vi "avg_spectrum_gen.vi"(0 "IR_off_q_in":refnum<queue>, 1 "IR_off_q_error_in":errorcluster, 2 "IR_on_q_in":refnum<queue>, 3 "IR_on_q_error_in":errorcluster, 4 "power_q_in":refnum<queue>, 5 "power_q_error_in":errorcluster, 6 "Number of sweeps":dbl) -> (7 "Avg Off Trace":waveform(dbl), 8 "Off queue length":i32, 9 "Avg On Trace":waveform(dbl), 10 "On queue length":i32, 11 "Difference Trace":waveform(dbl), 12 "Finished Gathering":bool, 13 "Avg Power / J":dbl format="%#_6f", 14 "IR_off_q_out":refnum<queue>, 15 "IR_off_q_error_out":errorcluster, 16 "IR_on_q_out":refnum<queue>, 17 "IR_on_q_error_out":errorcluster, 18 "power_q_out":refnum<queue>, 19 "power_q_error_out":errorcluster)   [LabVIEW 2020]
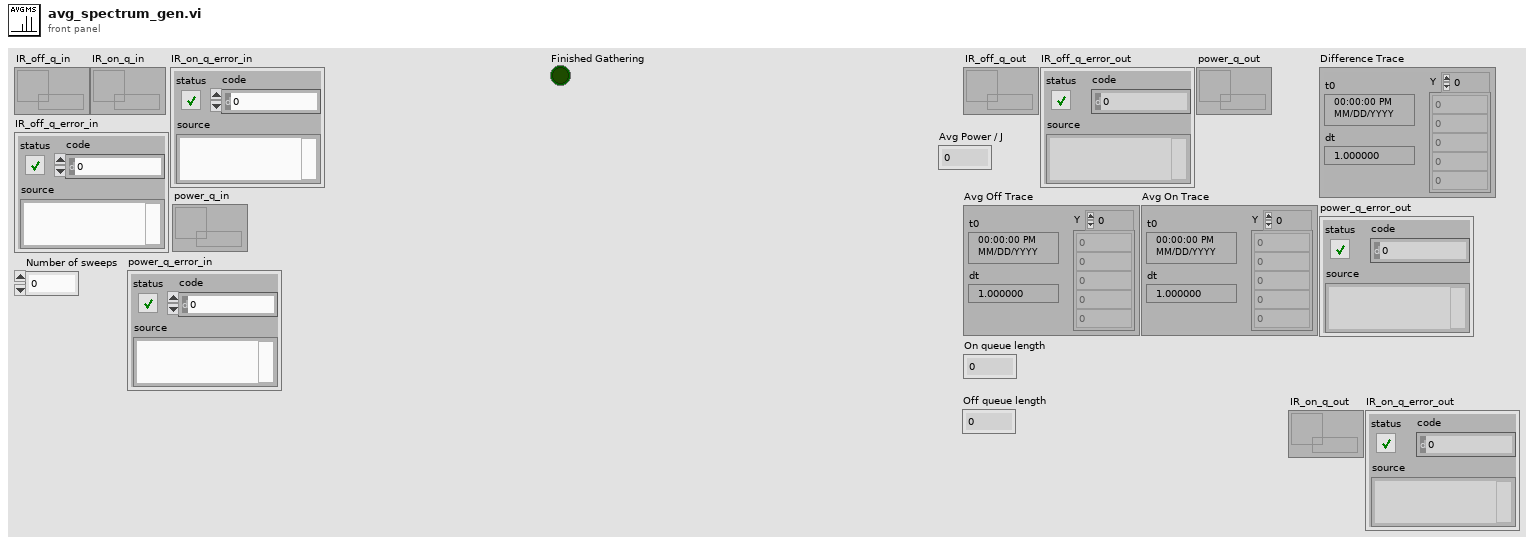
[diagram p1: front panel]
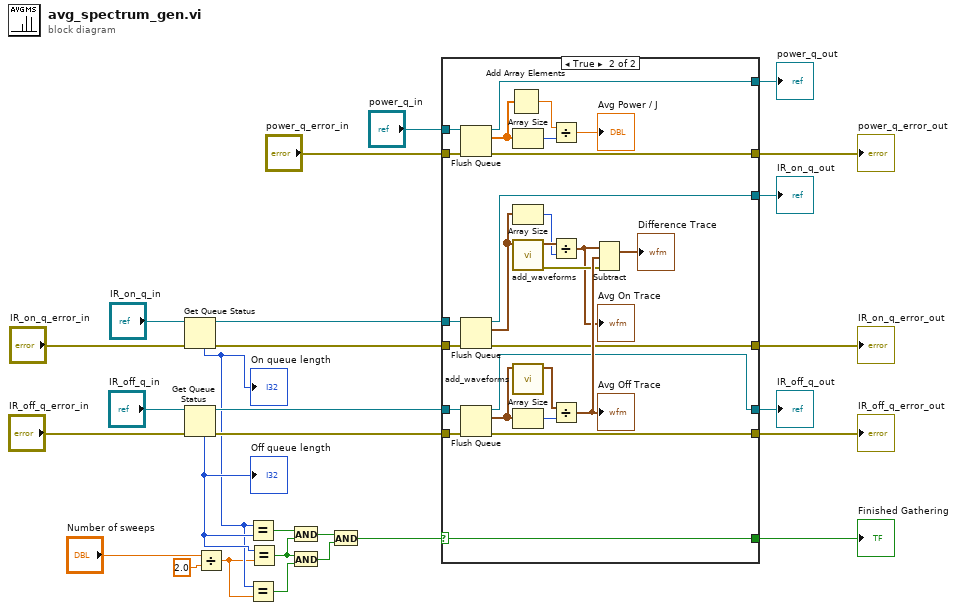
[diagram p0: block diagram]
diagram:
  n1 = Get Queue Status(queue="IR_on_q_in", error in (no error)="IR_on_q_error_in") -> (queue out=w24:refnum<queue>, error out=w23:errorcluster, # elements in queue=w14:i32)  [unwired: 1 in, 5 out]
  "On queue length" <- w14
  n2 = Get Queue Status(queue="IR_off_q_in", error in (no error)="IR_off_q_error_in") -> (queue out=w26:refnum<queue>, error out=w25:errorcluster, # elements in queue=w15:i32)  [unwired: 1 in, 5 out]
  "Off queue length" <- w15
  n3 = Divide(x="Number of sweeps", y=2.0) -> (x/y=w4:dbl)
  n4 = Equal?(x=w14, y=w15) -> (x = y?=w11:bool)
  n5 = Equal?(x=w14, y=w4) -> (x = y?=w9:bool)
  n6 = Equal?(x=w15, y=w4) -> (x = y?=w8:bool)
  n7 = And(x=w11, y=w8) -> (x .and. y?=w10:bool)
  n8 = And(x=w8, y=w9) -> (x .and. y?=w3:bool)
  n9 = And(x=w10, y=w3) -> (x .and. y?=w16:bool)
  n10 = case shown="True" w16 {
    selector: w16 -> [w31 w44]
    tunnel: w26 -> [w35 w62]
    tunnel: w25 -> [w34 w61]
    tunnel: w24 -> [w33 w60]
    tunnel: w23 -> [w32 w59]
    tunnel: [w35 w50] -> w20
    tunnel: [w34 w49] -> w19
    tunnel: [w33 w48] -> w18
    tunnel: [w32 w47] -> w17
    tunnel: [w31 w44] -> w7
    tunnel: "power_q_in" -> [w30 w43]
    tunnel: "power_q_error_in" -> [w29 w42]
    tunnel: [w30 w41] -> w6
    tunnel: [w29 w40] -> w5
    frame False {
    }
    frame True {
      n11 = Flush Queue(queue=w43, error in (no error)=w42) -> (queue out=w41:refnum<queue>, remaining elements=w39:dbl[], error out=w40:errorcluster)
      n12 = Flush Queue(queue=w60, error in (no error)=w59) -> (queue out=w48:refnum<queue>, remaining elements=w58:waveform(dbl)[], error out=w47:errorcluster)
      n13 = Flush Queue(queue=w62, error in (no error)=w61) -> (queue out=w50:refnum<queue>, remaining elements=w57:waveform(dbl)[], error out=w49:errorcluster)
      n14 = Add Array Elements(numeric array=w39) -> (sum=w38:dbl)
      n15 = Array Size(array=w39) -> (size(s)=w37:i32)
      n16 = Array Size(array=w58) -> (size(s)=w53:i32)
      n17 = call "add_waveforms.vi"("Waveform array"=w58) -> ("error out"=w51:errorcluster, "Waveform out"=w54:waveform(dbl))  [unwired: 9 in]
      n18 = call "add_waveforms.vi"("Waveform array"=w57) -> ("Waveform out"=w56:waveform(dbl))  [unwired: 9 in, 1 out]
      n19 = Array Size(array=w57) -> (size(s)=w55:i32)
      n20 = Divide(x=w38, y=w37) -> (x/y=→"Avg Power / J":dbl)
      n21 = Divide(x=w54, y=w53) -> (x/y=w46:waveform(dbl))
      "Avg On Trace" <- w46
      n22 = Divide(x=w56, y=w55) -> (x/y=w52:waveform(dbl))
      "Avg Off Trace" <- w52
      n23 = Subtract(1:w52, 2:w46, 4:w51) -> (0:→"Difference Trace":waveform(dbl))  [unwired: 1 out]
    }
  }
  "IR_off_q_out" <- w20
  "IR_off_q_error_out" <- w19
  "IR_on_q_out" <- w18
  "IR_on_q_error_out" <- w17
  "Finished Gathering" <- w7
  "power_q_out" <- w6
  "power_q_error_out" <- w5
